vi "Write Speaker.vi"(8 "error in (no error)":errorcluster, 10 "Speaker":T1, 11 "Reset cycle state STEP in":refnum<class "Reset cycle state STEP.lvclass">) -> (0 "error out":errorcluster, 3 "Reset cycle state STEP out":refnum<class "Reset cycle state STEP.lvclass">)   [LabVIEW 2014, in "Reset cycle state STEP.lvclass"]
uses:
  Reset cycle state STEP.lvclass
  Reset cycle state STEP.lvclass/Reset cycle state STEP.ctl
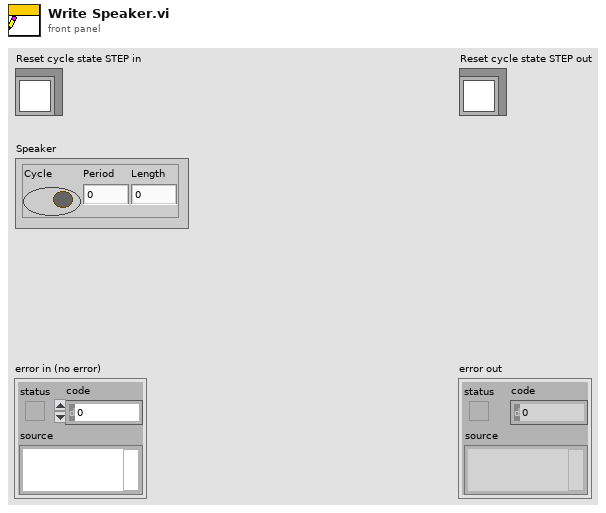
[diagram p1: front panel]
types:
  T1 = cluster{"Cycle":bool, "Period":i16, "Length":i16}
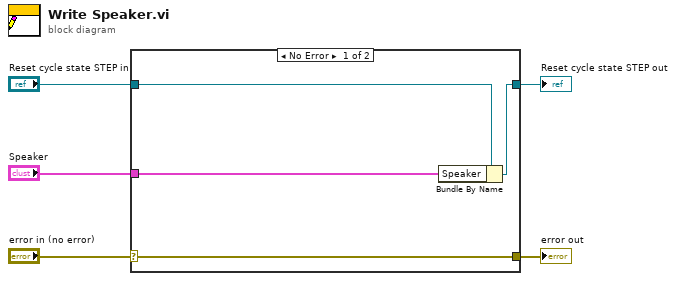
[diagram p0: block diagram]
diagram:
  n1 = case shown="No Error" "error in (no error)" {
    selector: "error in (no error)" -> [w9 w10]
    tunnel: [w9 w10] -> w4
    tunnel: [w7 w11] -> w2
    tunnel: "Reset cycle state STEP in" -> [w8 w11]
    tunnel: "Speaker" -> [w6 _]
    frame No Error {
      n2 = Bundle By Name(cluster=w8, "Speaker"=w6) -> (w7:refnum<class "Reset cycle state STEP.lvclass">)
    }
    frame Error {
    }
  }
  "error out" <- w4
  "Reset cycle state STEP out" <- w2
